vi "Constant fileExtension.vi"() -> (0 "Extension":string)   [LabVIEW 2018]
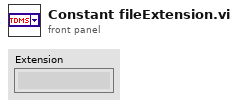
[diagram p1: front panel]
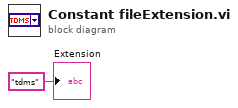
[diagram p0: block diagram]
diagram:
  "Extension" <- "tdms" ("String")
